vi "Measure - NI 9472.vi"(8 "Error In":errorcluster) -> (0 "Error Out":errorcluster)   [LabVIEW 2011]
uses:
  <vilib>/DAQmx/write.llb/DAQmx Write (Digital 1D U8 NChan 1Samp).vi
  <vilib>/DAQmx/miscellaneous.llb/DAQmx Fill In Error Info.vi
panel:
  in  "Stop Button":bool
  in  "Apply":bool
  in  "DIO States":bool[](array[boolean])=[FALSE, FALSE, FALSE, FALSE, FALSE, FALSE, FALSE, FALSE]
  out "DIO Leds":bool[](array[boolean])
  # "on"
  # "on"
  # "off"
  # "off"
  # "0        1         2         3        4         5         6        7"
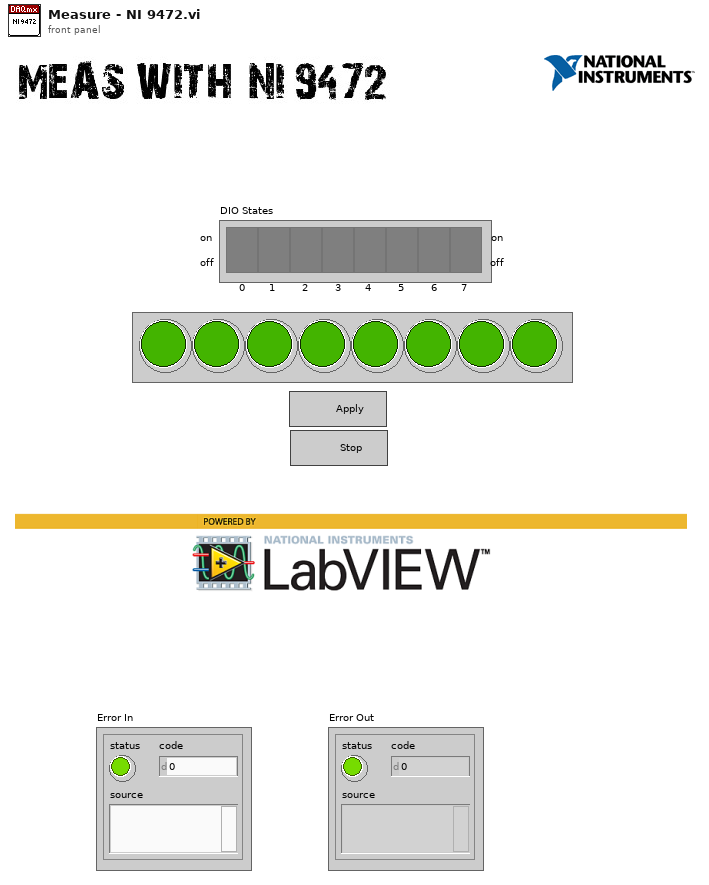
[diagram p1: front panel]
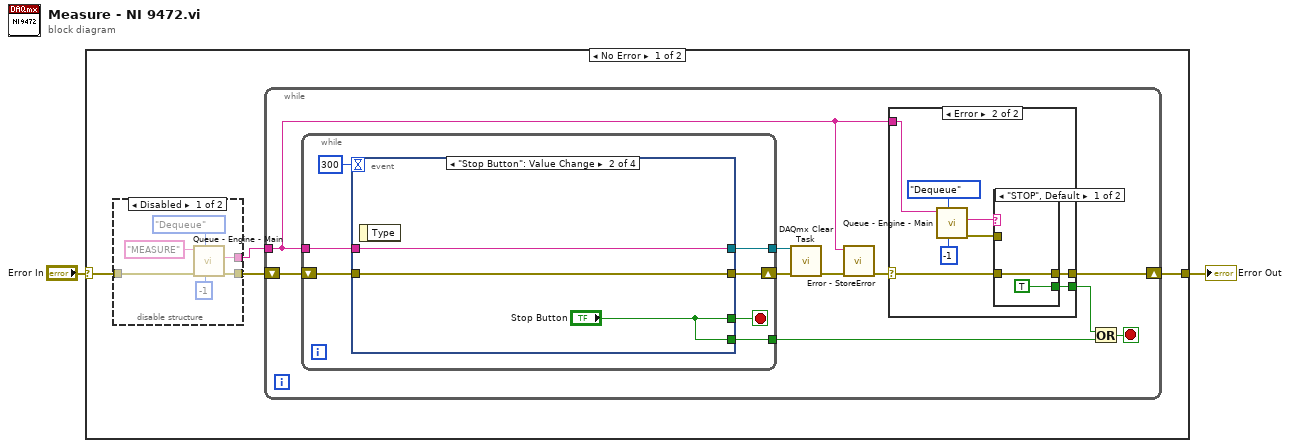
[diagram p0: block diagram]
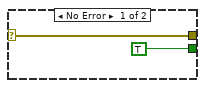
[diagram p2: hidden frame]
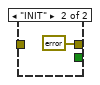
[diagram p3: hidden frame]
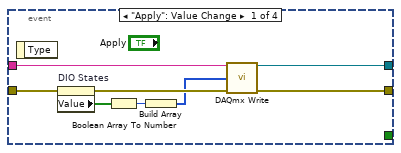
[diagram p4: hidden frame]
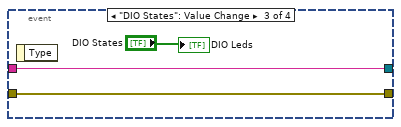
[diagram p5: hidden frame]
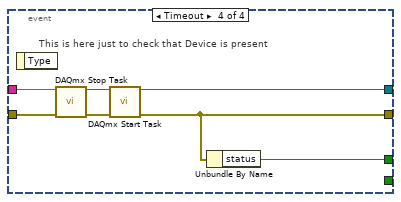
[diagram p6: hidden frame]
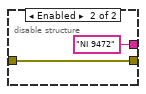
[diagram p7: hidden frame]
diagram:
  n1 = case shown="No Error" "Error In" {
    selector: "Error In" -> [w6 w66]
    tunnel: [w5 w66] -> w2
    frame No Error {
      n2 = disable-structure shown="Disabled" {
        disable-tunnel: [w63 w65] -> w3
        disable-tunnel: [w62 "NI 9472" ("Variable In")] -> w4
        disable-tunnel: w6 -> [w61 w65]
        frame Disabled {
          n3 = call "Queue - Engine - Main.vi"("timeout in ms (-1)"=-1, "Operation"=enum16{"Enqueue", "Dequeue", "Flush", "Release"}."Dequeue", "error in"=w61, "Queue Name In"="MEASURE") -> ("error out"=w63:errorcluster, "Data Out"=w62:string)  [unwired: 5 in, 1 out]
        }
        frame Enabled {
        }
      }
      n4 = while {
        tunnel: w4 -> [w7]
        shift-right: [w11] -> w5
        shift-left: w3 -> [w13]
        stop <- w8 stop-if-true
        n5 = while {
          tunnel: [w36] -> w16
          tunnel: w7 -> [w35]
          shift-right: [w34] -> w15
          shift-left: w13 -> [w33]
          tunnel: [w30] -> w9
          stop <- w32 stop-if-true
          n6 = event shown="[1] \"Stop Button\": Value Change" {
            selector: _ -> [_ _ _ _]
            dyn-events: _ -> [_ _ _ _]
            timeout: 300 -> [_ _ _ _]
            tunnel: [w44 w47 w50 w51] -> w36
            tunnel: w35 -> [w43 w47 w50 w55]
            tunnel: [w42 w46 w49 w52] -> w34
            tunnel: w33 -> [w39 w46 w49 w56]
            tunnel: [_ "Stop Button" _ w57] -> w32
            tunnel: [_ "Stop Button" _ _] -> w30
            event "Apply": Value Change {
              n7 = event-data() -> ()  [unwired: 1 in, 1 out]
              n8 = property on="DIO States" class="Arr (strict)"(error in=w39) -> (error out=w38:errorcluster, "Value"=w40:bool[])  [unwired: 1 in, 1 out]
              n9 = Boolean Array To Number(Boolean array=w40) -> (number=w41:u32)
              n10 = Build Array(w41) -> (w37:u32[])
              n11 = call-poly <vilib>:"DAQmx Write.vi"("task/channels in"=w43, "data"=w37, "error in"=w38) -> ("task out"=w44:refnum<k21>, "error out"=w42:errorcluster)  [unwired: 1 in, 10 out]
            }
            event "Stop Button": Value Change {
              n12 = event-data() -> ()  [unwired: 1 in, 1 out]
            }
            event "DIO States": Value Change {
              n13 = event-data() -> ()  [unwired: 1 in, 1 out]
              "DIO Leds" <- "DIO States"
            }
            event Timeout {
              # "This is here just to check that Device is present"
              n14 = event-data() -> ()  [unwired: 1 in, 1 out]
              n15 = call <vilib>:"DAQmx Stop Task.vi"("task/channels in"=w55, "error in"=w56) -> ("task out"=w54:refnum<k21>, "error out"=w53:errorcluster)  [unwired: 12 in]
              n16 = call <vilib>:"DAQmx Start Task.vi"("task/channels in"=w54, "error in"=w53) -> ("task out"=w51:refnum<k21>, "error out"=w52:errorcluster)  [unwired: 12 in]
              n17 = Unbundle By Name(w52) -> ("status"=w57:bool)
            }
          }
        }
        n18 = call <vilib>:"DAQmx Clear Task.vi"("task in"=w16, "error in"=w15) -> ("error out"=w14:errorcluster)  [unwired: 13 out]
        n19 = call "Error - StoreError.vi"("Error In"=w14, "Error Source In"=w7) -> ("Error Out"=w12:errorcluster)  [unwired: 8 in, 1 out]
        n20 = case shown="Error" w12 {
          selector: w12 -> [w18 w19]
          tunnel: [w18 w21] -> w11
          tunnel: [TRUE w20] -> w10
          tunnel: w7 -> [_ w24]
          frame No Error {
          }
          frame Error {
            n21 = call "Queue - Engine - Main.vi"("timeout in ms (-1)"=-1, "Operation"=enum16{"Enqueue", "Dequeue", "Flush", "Release"}."Dequeue", "Queue Name In"=w24) -> ("error out"=w23:errorcluster, "Data Out"=w22:string)  [unwired: 6 in, 1 out]
            n22 = case shown="\"STOP\", Default" w22 {
              tunnel: w23 -> [_ _]
              tunnel: [w27 errorcluster {"status"=FALSE, "code"=0, "source"=""} ("error out")] -> w21
              tunnel: [TRUE _] -> w20
              tunnel: w19 -> [w27 _]
              frame "STOP", Default {
              }
              frame "INIT" {
              }
            }
          }
        }
        n23 = Or(x=w10, y=w9) -> (x .or. y?=w8:bool)
      }
    }
    frame Error {
    }
  }
  "Error Out" <- w2
